vi "Arcade Drive.vi"(10 "Turn Power":dbl, 11 "Y Power":dbl) -> (2 "Right Motor Output":dbl, 3 "Left Motor Output":dbl)   [LabVIEW 2016]
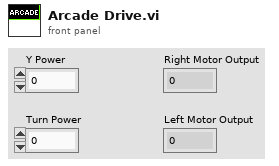
[diagram p1: front panel]
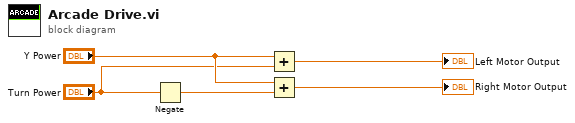
[diagram p0: block diagram]
diagram:
  n1 = Negate(x="Turn Power") -> (-x=w2:dbl)
  n2 = Add(x="Y Power", y="Turn Power") -> (x+y=→"Left Motor Output":dbl)
  n3 = Add(x="Y Power", y=w2) -> (x+y=→"Right Motor Output":dbl)
